vi "AreWeInTransition.vi"(11 "Last Commanded Sailing Regime":T1) -> (3 "Are We In Transition?":bool)   [LabVIEW 2013]
doc: "This VI checks the past regime and checks whether we were in a transition. If so, the code will check whether the transistion has either failed or completed, and stays in transition otherwise. This is done to make sure a commanded transition goes to completion or failure instead rechecking every cycle whether the transition should be recommanded.\n\nEric Schneider, Feb. 2014"
uses:
  Data/TypeDefs/Sailing Regimes.ctl
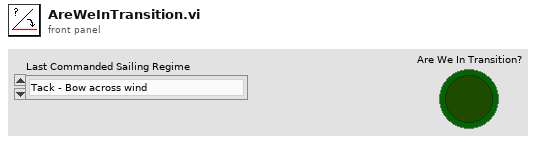
[diagram p1: front panel]
types:
  T1 = typedef "Sailing Regimes.ctl" = enum16{"Tack - Bow across wind", "Upwind - Starboard Tack", "Turn between Upwind/Reach - Starboard Tack", "Reach - Starboard Tack", "Turn between Reach/Run - Starboard Tack", "Run - Starboard Tack", "Jibe - Stern across wind", "Run - Port Tack", "Turn between Reach/Run - Port Tack", "Reach - Port Tack", "Turn between Upwind/Reach - Port Tack", "Upwind - Port Tack"}
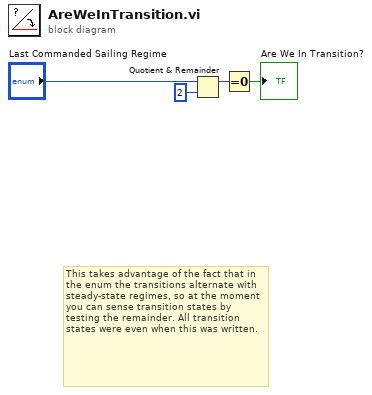
[diagram p0: block diagram]
diagram:
  # "This takes advantage of the fact that in the enum the transitions alternate with steady-state regimes, so at the moment you can sense transition states by testing the remainder. All transition states were even when this was written."
  n1 = Quotient & Remainder(x="Last Commanded Sailing Regime", y=2) -> (x-y*floor(x/y)=w2:i32)  [unwired: 1 out]
  n2 = Equal To 0?(x=w2) -> (x = 0?=→"Are We In Transition?":bool)
